vi "template-state-machine-basic.vi"() -> ()   [LabVIEW 2024]
uses:
  state-enum.ctl
  utils-sub-vi/csv-file-logging-util/filepath-selection.ctl
  utils-sub-vi/csv-file-logging-util/datalogging-options.ctl
  serial-options.ctl
  sensor-options.ctl
panel:
  out "return count":u32
  out "Bytes at Port":u32
  out "Log File Open":bool
  in  "Tab Control":enum32{"Data", "Settings"}(tab)
  in  "?":dbl(slide) scale=0.0..10.0
  out "Logged CSV out":string
  out "Serial msg":string
  in  "Datalogging options":T1={"data-precision"=3, "Include Date"=FALSE, "Include Timestamp"=TRUE, "Include Milliseconds"=FALSE, "sample-rate (Hz)"=4.0, "Logging Active"=TRUE}
  in  "Log Filepath Selection":T2={"Log Filepath Source"=enum."Application Relative (Auto)", "Log File Path (Manual)"=path "C:/Users/dheard/Documents/0002-labview-projects/adam-4xxx/template/data", "Log File Folder Name"="data", "log file name"="log", "Include Date in Filename"=TRUE, "Include Time in Filename"=TRUE}
  in  "Serial Port Options":T3={"COM Port (COM10)"="COM10", "baud rate (19200)"=19200, "Simulate Hardware"=FALSE} {"baud rate (19200)" max=115200 step=1200}
  in  "Sensor Options":T4={"Display Units"="PSI", "Zero Offset"=2.62, "Sensor Min"=0.0, "Sensor Max"=500.0, "Signal Min"=0.0, "Signal Max"=100.0, "Conversion Factor"=0.0}
  in  "save-settings":bool
  in  "load-settings":bool
  in  "Settings file":path
  out "Sample Rate (Hz)":dbl format="%-#3.3f"
  in  "Debug Mode":bool
  out "Loop Time (mS)":u32
  out "State:":T5
  out "error IO":errorcluster
  in  "stop":bool
  in  "start":bool
  in  "Exit":bool
  # "Template Logger"
  # "Conversion Factor to\nCalculate User Units from Sensor Units"
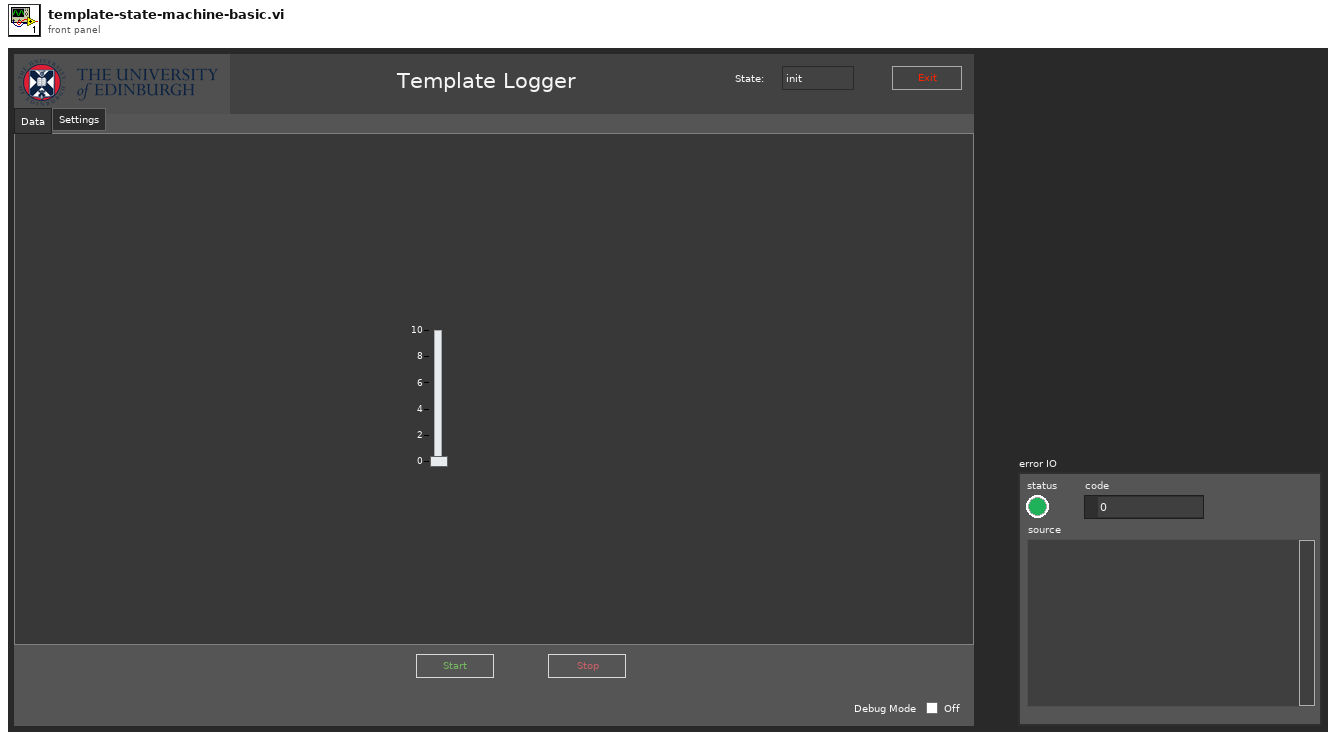
[diagram p1: front panel]
types:
  T1 = typedef "datalogging-options.ctl" = cluster{"data-precision":i32, "Include Date":bool, "Include Timestamp":bool, "Include Milliseconds":bool, "sample-rate (Hz)":dbl, "Logging Active":bool}
  T2 = typedef "filepath-selection.ctl" = cluster{"Log Filepath Source":enum16{"Application Relative (Auto)", "VI Relative (Auto)", "Complete Path (Manual)"}, "Log File Path (Manual)":path, "Log File Folder Name":string, "log file name":string, "Include Date in Filename":bool, "Include Time in Filename":bool}
  T3 = typedef "serial-options.ctl" = cluster{"COM Port (COM10)":refnum<visa-resource-name>, "baud rate (19200)":u32, "Simulate Hardware":bool}
  T4 = typedef "sensor-options.ctl" = cluster{"Display Units":string, "Zero Offset":dbl, "Sensor Min":dbl, "Sensor Max":dbl, "Signal Min":dbl, "Signal Max":dbl, "Conversion Factor":dbl}
  T5 = typedef "state-enum.ctl" = enum16{"init", "recall-settings", "save-settings", "wait", "start", "pre-run", "run", "stop", "shutdown", "exit"}
  T6 = enum8{"Enabled", "Disabled", "Disabled and Grayed Out"}
  T7 = enum16{"open", "replace", "create", "open or create", "replace or create", "replace or create with confirmation"}
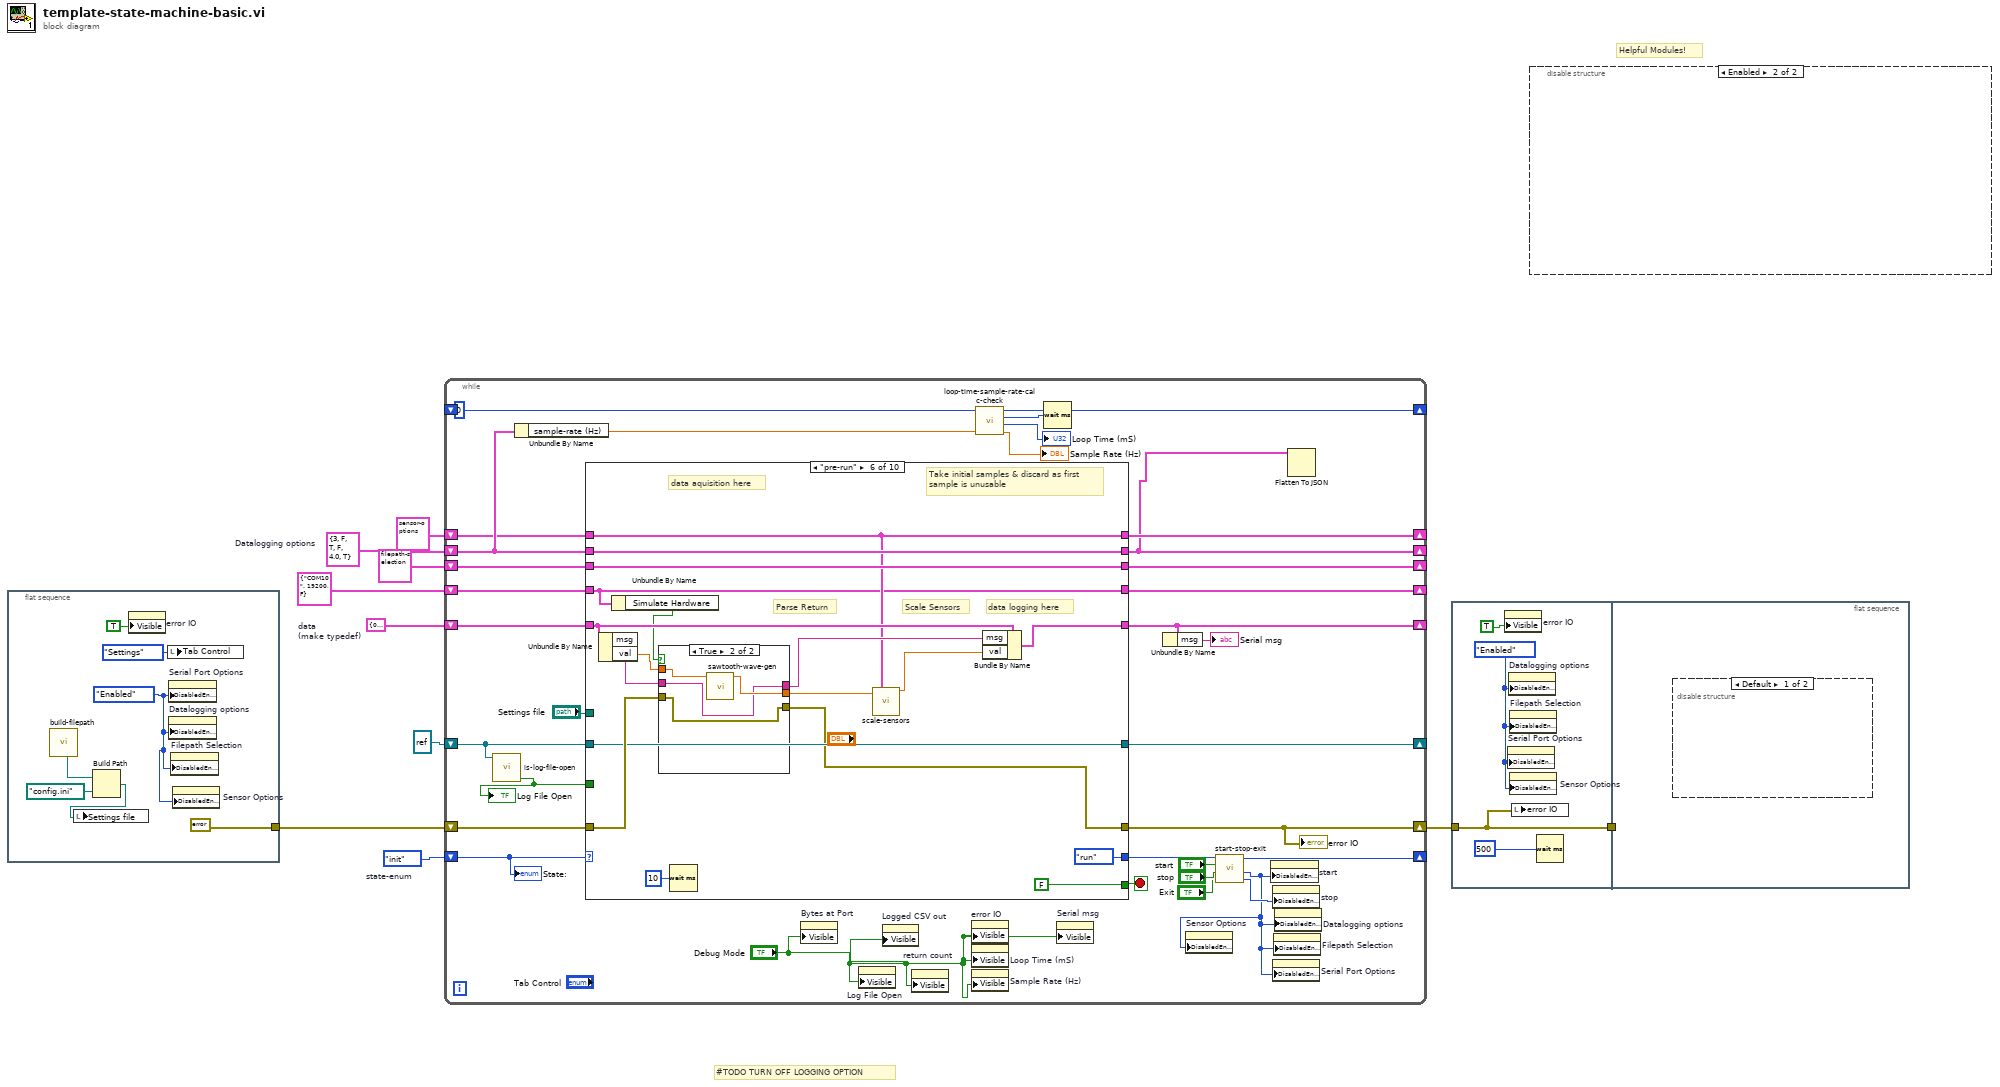
[diagram p0: block diagram]
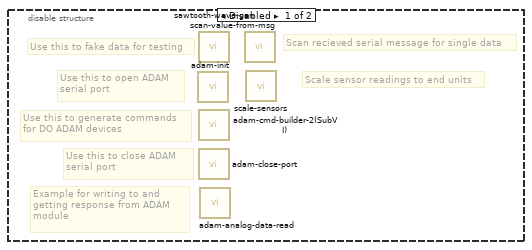
[diagram p2: hidden frame]
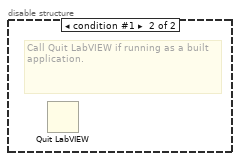
[diagram p3: hidden frame]
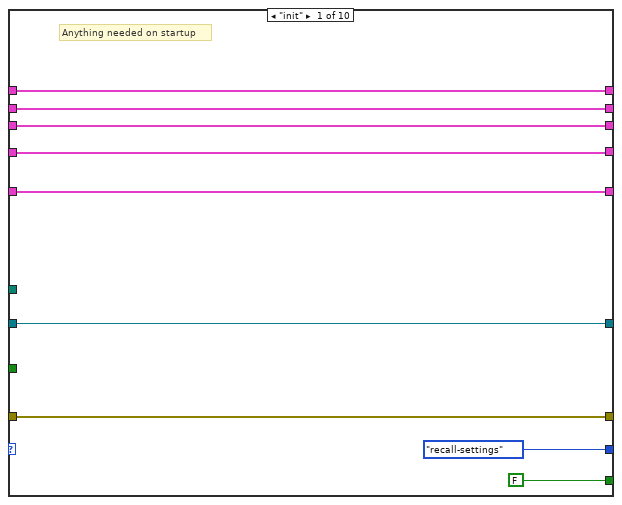
[diagram p4: hidden frame]
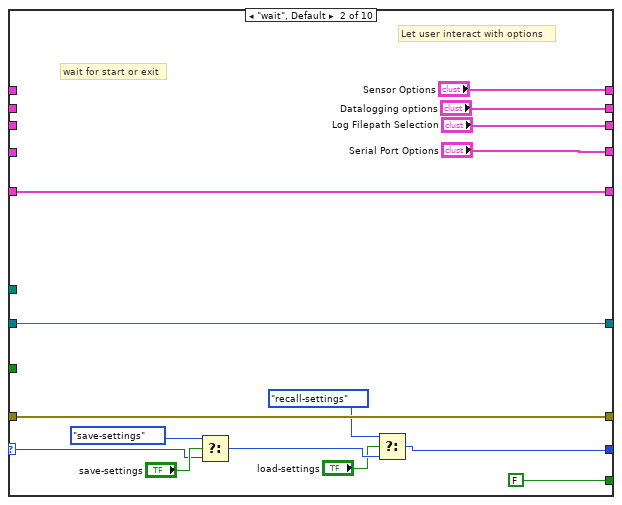
[diagram p5: hidden frame]
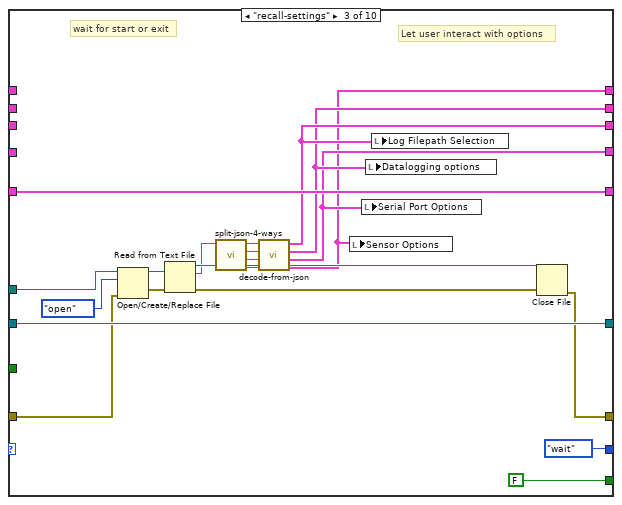
[diagram p6: hidden frame]
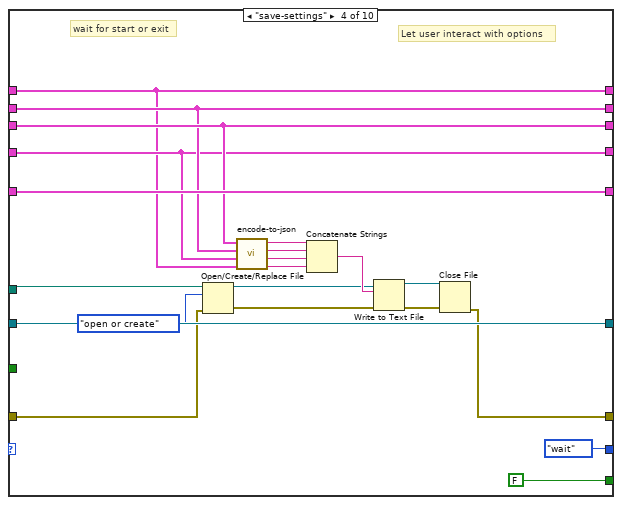
[diagram p7: hidden frame]
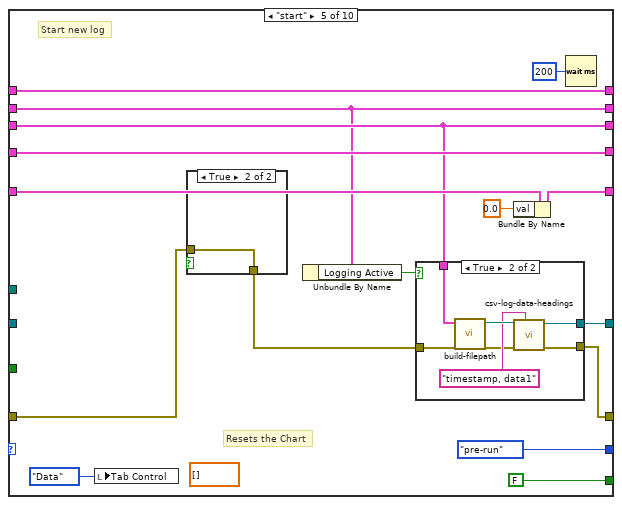
[diagram p8: hidden frame]
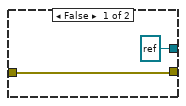
[diagram p10: hidden frame]
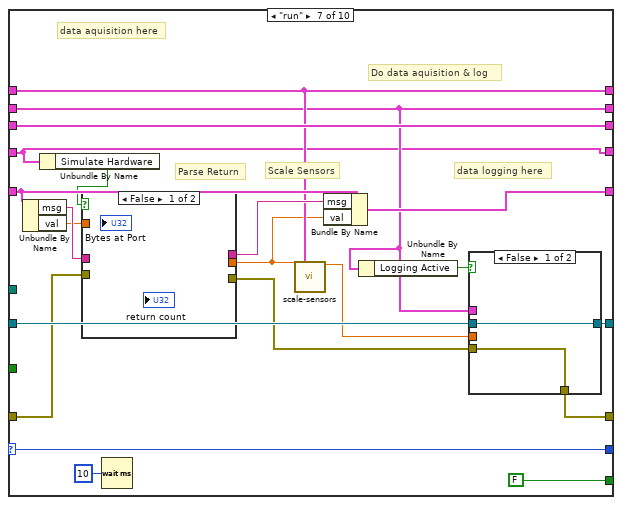
[diagram p12: hidden frame]
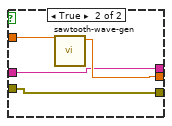
[diagram p13: hidden frame]
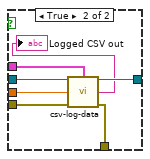
[diagram p14: hidden frame]
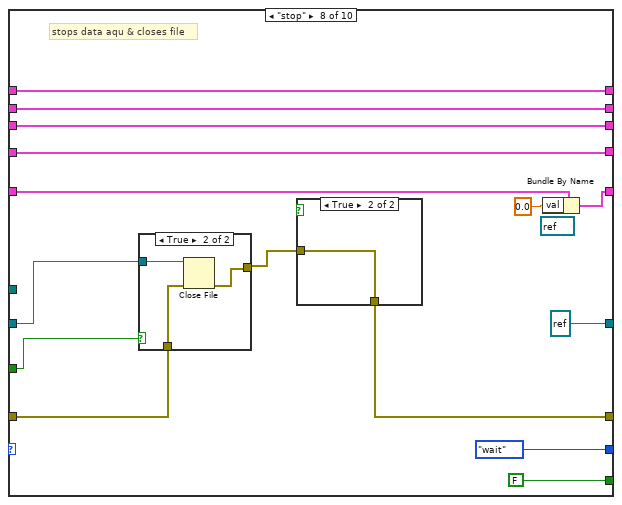
[diagram p15: hidden frame]
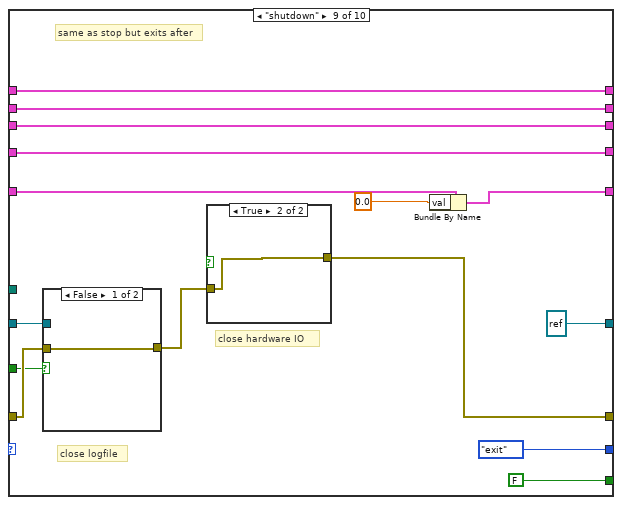
[diagram p18: hidden frame]
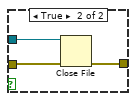
[diagram p20: hidden frame]
diagram:
  w3 = T1 {"data-precision"=3, "Include Date"=FALSE, "Include Timestamp"=TRUE, "Include Milliseconds"=FALSE, "sample-rate (Hz)"=4.0, "Logging Active"=TRUE}  # Datalogging options
  w8 = cluster{"val":dbl, "bool":bool, "msg":string} {"val"=0.0, "bool"=FALSE, "msg"=""}  # data (make typedef)
  w11 = state-enum."init"  # state-enum
  # "#TODO TURN OFF LOGGING OPTION"
  # "Helpful Modules!"
  n1 = flat-sequence {
    tunnel: [errorcluster {"status"=FALSE, "code"=0, "source"=""} ("error IO")] -> w7
    frame #0 {
      w15 = T6."Enabled" ("Disabled")
      n2 = call "build-filepath.vi"() -> ("Application Directory"=w14:path)  [unwired: 9 in, 2 out]
      n3 = Build Path(base path=w14, name or relative path=path "config.ini") -> (appended path=w12:path)
      n4 = local write "Settings file"(w12) -> ()
      n5 = property on="error IO" class="Clust (strict)"("Visible"=TRUE) -> ()  [unwired: 2 in, 2 out]
      n6 = local write "Tab Control"(enum32{"Data", "Settings"}."Settings" ("Tab Control")) -> ()
      n7 = property on="Serial Port Options" class="Clust (strict)"("DisabledEnum"=w15) -> ()  [unwired: 2 in, 2 out]
      n8 = property on="Datalogging options" class="Clust (strict)"("DisabledEnum"=w15) -> ()  [unwired: 2 in, 2 out]
      n9 = property on="Filepath Selection" class="Clust (strict)"("DisabledEnum"=w15) -> ()  [unwired: 2 in, 2 out]
      n10 = property on="Sensor Options" class="Clust (strict)"("DisabledEnum"=w15) -> ()  [unwired: 2 in, 2 out]
    }
  }
  n11 = while {
    shift-right: [w49] -> _
    shift-left: w11 -> [w51]
    shift-right: [w43] -> w9
    shift-left: w7 -> [w44]
    shift-right: [w26] -> _
    shift-left: w8 -> [w42]
    shift-right: [w39] -> _
    shift-left: u32 0 ("millisecond timer value") -> [w41]
    shift-right: [w35] -> _
    shift-left: T2 {"Log Filepath Source"=enum."Application Relative (Auto)", "Log File Path (Manual)"=path "C:/Users/dheard/Documents/0002-labview-projects/ammonia-absorbsion-rig/data", "Log File Folder Name"="data", "log file name"="log", "Include Date in Filename"=TRUE, "Include Time in Filename"=TRUE} ("Filepath Selection") -> [w34]
    shift-right: [w33] -> _
    shift-left: refnum<file> refnum ("Byte Stream File out") -> [w32]
    shift-right: [w20] -> _
    shift-left: w3 -> [w30]
    shift-right: [w27] -> _
    shift-left: T3 {"COM Port (COM10)"="COM10", "baud rate (19200)"=19200, "Simulate Hardware"=FALSE} ("Serial Port Options") -> [w28]
    shift-right: [w24] -> _
    shift-left: T4 {"Display Units"="units", "Zero Offset"=2.62, "Sensor Min"=0.0, "Sensor Max"=500.0, "Signal Min"=0.0, "Signal Max"=100.0, "Conversion Factor"=0.0} ("Sensor Options") -> [w22]
    stop <- w45 stop-if-true
    n12 = call "is-log-file-open.vi"("Byte Stream File in"=w32) -> ("Log File Open"=w31:bool)  [unwired: 10 in]
    "Log File Open" <- w31
    n13 = Unbundle By Name(w30) -> ("sample-rate (Hz)"=w29:dbl)
    n14 = case shown="\"pre-run\"" w51 {
      selector: w51 -> [_ w66 _ _ _ _ w185 _ _ _]
      tunnel: [state-enum."recall-settings" w61 state-enum."wait" state-enum."wait" state-enum."pre-run" state-enum."run" w185 state-enum."wait" state-enum."exit" state-enum."exit"] -> w50
      tunnel: [FALSE FALSE FALSE FALSE FALSE FALSE FALSE FALSE FALSE TRUE] -> w45
      tunnel: [w58 w74 w86 w97 w127 w149 w180 w202 w222 w248] -> w43
      tunnel: w44 -> [w58 w74 w90 w103 w124 w157 w179 w207 w228 w248]
      tunnel: [w57 w73 w95 w116 w130 w160 w184 w210 w231 w247] -> w26
      tunnel: w42 -> [w57 w73 w95 w116 w131 w155 w177 w212 w233 w247]
      tunnel: [w55 "Log Filepath Selection" w79 w110 w120 w159 w181 w206 w227 w245] -> w35
      tunnel: w34 -> [w55 _ _ w110 w120 w159 w181 w206 w227 w245]
      tunnel: [w56 w71 w94 w115 w128 w150 w182 refnum<file> refnum ("log file Byte Stream File out") refnum<file> refnum ("log file Byte Stream File out") w246] -> w33
      tunnel: w32 -> [w56 w71 w94 w115 _ w150 w183 w209 w230 w246]
      tunnel: [w54 "Datalogging options" w78 w109 w119 w158 w171 w205 w226 w244] -> w20
      tunnel: w30 -> [w54 _ _ w109 w119 w158 w171 w205 w226 w244]
      tunnel: w31 -> [_ _ _ _ _ _ _ w200 w225 _]
      tunnel: w28 -> [w53 _ _ w108 w125 w146 w169 w204 w224 w243]
      tunnel: [w53 "Serial Port Options" w77 w108 w125 w146 w169 w204 w224 w243] -> w27
      tunnel: [w52 "Sensor Options" w76 w107 w122 w152 w173 w201 w221 w242] -> w24
      tunnel: w22 -> [w52 _ _ w107 w122 w152 w173 w201 w221 w242]
      tunnel: "Settings file" -> [_ _ w92 w98 _ _ _ _ _ _]
      frame "init" {
        # "Anything needed on startup"
      }
      frame "wait", Default {
        # "Let user interact with options"
        # "wait for start or exit"
        n15 = Select(t=state-enum."save-settings", s="save-settings", f=w66) -> (s? t:f=w64:T5)
        n16 = Select(t=state-enum."recall-settings", s="load-settings", f=w64) -> (s? t:f=w61:T5)
      }
      frame "recall-settings" {
        # "Let user interact with options"
        # "wait for start or exit"
        n17 = Open/Create/Replace File(file path (use dialog)=w92, error in=w90, operation (0:open)=T7."open") -> (refnum out=w89:refnum<file>, error out=w88:errorcluster)  [unwired: 3 in, 1 out]
        n18 = Read from Text File(file (use dialog)=w89, error in=w88) -> (refnum out=w85:refnum<file>, text=w84:string, error out=w87:errorcluster)  [unwired: 2 in, 1 out]
        n19 = call "split-json-4-ways.vi"("json-string-in"=w84) -> ("sensor-json"=w80:string, "serial-json"=w81:string, "datalogging-json"=w82:string, "filepath-json"=w83:string)  [unwired: 7 in]
        n20 = call "decode-from-json.vi"("sensor-options-json"=w80, "serial-port-json"=w81, "data-logging-json"=w82, "filepath-json"=w83) -> ("Sensor Option Recall"=w76:T4, "Serial Port Recall"=w77:T3, "Datalogging Recall"=w78:T1, "Filepath Recall"=w79:T2)  [unwired: 4 in]
        n21 = local write "Sensor Options"(w76) -> ()
        n22 = local write "Serial Port Options"(w77) -> ()
        n23 = local write "Datalogging options"(w78) -> ()
        n24 = local write "Log Filepath Selection"(w79) -> ()
        n25 = Close File(refnum=w85, error in=w87) -> (error out=w86:errorcluster)  [unwired: 1 out]
      }
      frame "save-settings" {
        # "Let user interact with options"
        # "wait for start or exit"
        n26 = Open/Create/Replace File(file path (use dialog)=w98, error in=w103, operation (0:open)=T7."open or create") -> (refnum out=w102:refnum<file>, error out=w101:errorcluster)  [unwired: 3 in, 1 out]
        n27 = call "encode-to-json.vi"("Sensor Options"=w107, "Serial Port Options"=w108, "Datalogging options"=w109, "Filepath Selection"=w110) -> ("sensor-options-json"=w106:string, "serial-port-json"=w111:string, "data-logging-json"=w112:string, "filepath-json"=w113:string)  [unwired: 4 in]
        n28 = Concatenate Strings(w113, w112, w111, w106) -> (w105:string)
        n29 = Write to Text File(file (use dialog)=w102, text=w105, error in=w101) -> (refnum out=w100:refnum<file>, error out=w99:errorcluster)  [unwired: 1 in, 1 out]
        n30 = Close File(refnum=w100, error in=w99) -> (error out=w97:errorcluster)  [unwired: 1 out]
      }
      frame "start" {
        (unwired) dbl[] [] ("History Data")
        # "Start new log"
        # "Resets the Chart"
        n31 = local write "Tab Control"(enum32{"Data", "Settings"}."Data" ("Tab Control")) -> ()
        n32 = case shown="True" {
          selector: _ -> [_ _]
          tunnel: w124 -> [w134 w135]
          tunnel: [w134 w135] -> w123
          frame False {
          }
          frame True {
          }
        }
        n33 = Unbundle By Name(w119) -> ("Logging Active"=w118:bool)
        n34 = case shown="True" w118 {
          tunnel: [refnum<file> refnum ("Byte Stream File out") w141] -> w128
          tunnel: [w136 w140] -> w127
          tunnel: w123 -> [w136 w139]
          tunnel: w120 -> [_ w138]
          frame False {
          }
          frame True {
            n35 = call "build-filepath.vi"("Filepath Selection"=w138) -> ("appended path for log file"=w143:path)  [unwired: 8 in, 2 out]
            n36 = call "csv-log-data-headings.vi"("CSV Data Headings"="timestamp, data1", "error in (no error)"=w139, "Log File Path"=w143) -> ("error out"=w140:errorcluster, "Byte Stream File out"=w141:refnum<file>)  [unwired: 6 in, 1 out]
          }
        }
        n37 = Bundle By Name(cluster=w131, "val"=0.0 ("output")) -> (w130:cluster{"val":dbl, "bool":bool, "msg":string})
        n38 = Wait (ms)(milliseconds to wait=u32 200) -> ()  [unwired: 1 out]
      }
      frame "pre-run" {
        # "Take initial samples & discard as first\nsample is unusable"
        # "Scale Sensors"
        # "Parse Return"
        # "data logging here"
        # "data aquisition here"
        n39 = Unbundle By Name(w155) -> ("msg"=w154:string, "val"=w144:dbl)
        n40 = Unbundle By Name(w146) -> ("Simulate Hardware"=w145:bool)
        n41 = case shown="True" w145 {
          tunnel: w157 -> [_ w162]
          tunnel: w154 -> [_ w163]
          tunnel: [_ w163] -> w153
          tunnel: [_ w164] -> w151
          tunnel: [_ w162] -> w149
          tunnel: w144 -> [_ w165]
          frame False {
          }
          frame True {
            n42 = call "sawtooth-wave-gen.vi"("current-val"=w165) -> ("output"=w164:dbl)  [unwired: 10 in]
          }
        }
        n43 = Wait (ms)(milliseconds to wait=u32 10) -> ()  [unwired: 1 out]
        n44 = call "scale-sensors.vi"("Measured Value (mV)"=w151, "Sensor Options"=w152) -> ("Calculated Value (User Specified Unit)"=w147:dbl)  [unwired: 8 in, 5 out]
        n45 = Bundle By Name(cluster=w155, "msg"=w153, "val"=w147) -> (w160:cluster{"val":dbl, "bool":bool, "msg":string})
      }
      frame "run" {
        # "Scale Sensors"
        # "Parse Return"
        # "data logging here"
        # "data aquisition here"
        # "Do data aquisition & log"
        n46 = Unbundle By Name(w177) -> ("msg"=w176:string, "val"=w167:dbl)
        n47 = Unbundle By Name(w169) -> ("Simulate Hardware"=w168:bool)
        n48 = case shown="False" w168 {
          tunnel: w179 -> [_ w190]
          tunnel: w176 -> [_ w187]
          tunnel: [_ w190] -> w175
          tunnel: [_ w187] -> w174
          tunnel: [_ w188] -> w166
          tunnel: w167 -> [_ w189]
          frame False {
          }
          frame True {
            n49 = call "sawtooth-wave-gen.vi"("current-val"=w189) -> ("output"=w188:dbl)  [unwired: 10 in]
          }
        }
        n50 = Wait (ms)(milliseconds to wait=u32 10) -> ()  [unwired: 1 out]
        n51 = call "scale-sensors.vi"("Measured Value (mV)"=w166, "Sensor Options"=w173) -> ("Calculated Value (User Specified Unit)"=w172:dbl)  [unwired: 8 in, 5 out]
        n52 = Bundle By Name(cluster=w177, "msg"=w174, "val"=w166) -> (w184:cluster{"val":dbl, "bool":bool, "msg":string})
        n53 = Unbundle By Name(w171) -> ("Logging Active"=w170:bool)
        n54 = case shown="False" w170 {
          tunnel: w183 -> [w192 w199]
          tunnel: [w192 w198] -> w182
          tunnel: [w191 w196] -> w180
          tunnel: w171 -> [_ w195]
          tunnel: w175 -> [w191 w194]
          tunnel: w172 -> [_ w193]
          frame False {
          }
          frame True {
            n55 = call "csv-log-data.vi"("log file Byte Stream File in"=w199, "Datalogging options"=w195, "Data Point In"=w193, "error in (no error)"=w194) -> ("log file Byte Stream File out"=w198:refnum<file>, "Logged CSV out"=→"Logged CSV out":string, "error out"=w196:errorcluster)  [unwired: 7 in, 2 out]
          }
        }
      }
      frame "stop" {
        (unwired) refnum<visa-resource-name> refnum ("VISA resource name out")
        # "stops data aqu & closes file"
        n56 = case shown="True" w200 {
          tunnel: w209 -> [_ w220]
          tunnel: w207 -> [w217 w219]
          tunnel: [w217 w218] -> w203
          frame False {
          }
          frame True {
            n57 = Close File(refnum=w220, error in=w219) -> (error out=w218:errorcluster)  [unwired: 1 out]
          }
        }
        n58 = case shown="True" {
          selector: _ -> [_ _]
          tunnel: w203 -> [w215 w216]
          tunnel: [w215 w216] -> w202
          frame False {
          }
          frame True {
          }
        }
        n59 = Bundle By Name(cluster=w212, "val"=0.0 ("output")) -> (w210:cluster{"val":dbl, "bool":bool, "msg":string})
      }
      frame "shutdown" {
        # "close hardware IO"
        # "close logfile"
        # "same as stop but exits after"
        n60 = case shown="False" w225 {
          tunnel: w230 -> [_ w241]
          tunnel: w228 -> [w238 w240]
          tunnel: [w238 w239] -> w223
          frame False {
          }
          frame True {
            n61 = Close File(refnum=w241, error in=w240) -> (error out=w239:errorcluster)  [unwired: 1 out]
          }
        }
        n62 = case shown="True" {
          selector: _ -> [_ _]
          tunnel: w223 -> [w236 w237]
          tunnel: [w236 w237] -> w222
          frame False {
          }
          frame True {
          }
        }
        n63 = Bundle By Name(cluster=w233, "val"=0.0 ("output")) -> (w231:cluster{"val":dbl, "bool":bool, "msg":string})
      }
      frame "exit" {
        # "Exit safely"
      }
    }
    "error IO" <- w43
    n64 = property on="Bytes at Port" class="DigNum (strict)"("Visible"="Debug Mode") -> ()  [unwired: 2 in, 2 out]
    n65 = property on="Log File Open" class="Bool (strict)"("Visible"="Debug Mode") -> ()  [unwired: 2 in, 2 out]
    n66 = property on="Logged CSV out" class="Str"("Visible"="Debug Mode") -> ()  [unwired: 2 in, 2 out]
    n67 = property on="return count" class="DigNum (strict)"("Visible"="Debug Mode") -> ()  [unwired: 2 in, 2 out]
    n68 = property on="error IO" class="Clust (strict)"("Visible"="Debug Mode") -> ()  [unwired: 2 in, 2 out]
    n69 = property on="Loop Time (mS)" class="DigNum (strict)"("Visible"="Debug Mode") -> ()  [unwired: 2 in, 2 out]
    n70 = property on="Sample Rate (Hz)" class="DigNum (strict)"("Visible"="Debug Mode") -> ()  [unwired: 2 in, 2 out]
    n71 = call "loop-time-sample-rate-calc-check.vi"("sample-rate-Hz"=w29, "millisecond timer value in"=w41) -> ("Loop Hz"=→"Sample Rate (Hz)":dbl, "Loop Time (mS)"=→"Loop Time (mS)":u32, "sample-rate-delay-mS"=w36:u32, "millisecond timer value out"=w39:u32)  [unwired: 6 in]
    n72 = Wait (ms)(milliseconds to wait=w36) -> ()  [unwired: 1 out]
    n73 = property on="Serial msg" class="Str"("Visible"="Debug Mode") -> ()  [unwired: 2 in, 2 out]
    n74 = Unbundle By Name(w26) -> ("msg"=→"Serial msg":string)
    n75 = call "start-stop-exit.vi"("Exit"="Exit", "stop"="stop", "start"="start", "current-state"=w50) -> ("stop-enable"=w40:T6, "start-enable"=w23:T6, "new-state"=w49:T5)  [unwired: 5 in]
    n76 = property on="Sensor Options" class="Clust (strict)"("DisabledEnum"=w23) -> ()  [unwired: 2 in, 2 out]
    n77 = property on="start" class="Bool"("DisabledEnum"=w23) -> ()  [unwired: 2 in, 2 out]
    n78 = property on="stop" class="Bool"("DisabledEnum"=w40) -> ()  [unwired: 2 in, 2 out]
    n79 = property on="Serial Port Options" class="Clust (strict)"("DisabledEnum"=w23) -> ()  [unwired: 2 in, 2 out]
    n80 = property on="Filepath Selection" class="Clust (strict)"("DisabledEnum"=w23) -> ()  [unwired: 2 in, 2 out]
    n81 = property on="Datalogging options" class="Clust (strict)"("DisabledEnum"=w23) -> ()  [unwired: 2 in, 2 out]
    n82 = Flatten To JSON(anything=w20) -> ()  [unwired: 2 in, 2 out]
    "State:" <- w51
  }
  n83 = flat-sequence {
    tunnel: [w252] -> w10
    tunnel: w9 -> [w252]
    tunnel: w10 -> [_]
    frame #0 {
      w251 = T6."Enabled" ("Disabled")
      n84 = property on="error IO" class="Clust (strict)"("Visible"=TRUE) -> ()  [unwired: 2 in, 2 out]
      n85 = property on="Serial Port Options" class="Clust (strict)"("DisabledEnum"=w251) -> ()  [unwired: 2 in, 2 out]
      n86 = property on="Datalogging options" class="Clust (strict)"("DisabledEnum"=w251) -> ()  [unwired: 2 in, 2 out]
      n87 = property on="Filepath Selection" class="Clust (strict)"("DisabledEnum"=w251) -> ()  [unwired: 2 in, 2 out]
      n88 = property on="Sensor Options" class="Clust (strict)"("DisabledEnum"=w251) -> ()  [unwired: 2 in, 2 out]
      n89 = local write "error IO"(w252) -> ()
      n90 = Wait (ms)(milliseconds to wait=u32 500) -> ()  [unwired: 1 out]
    }
    frame #1 {
      n91 = disable-structure "Conditional Disable Structure" shown="Default" {
        frame condition #0 (active) {
        }
        frame condition #1 {
          # "Call Quit LabVIEW if running as a built application."
          n92 = Quit LabVIEW() -> ()  [unwired: 1 in]
        }
      }
    }
  }
  n93 = disable-structure shown="Enabled" {
    frame Disabled {
      # "Scale sensor readings to end units"
      # "Scan recieved serial message for single data"
      # "Example for writing to and\ngetting response from ADAM\nmodule"
      # "Use this to open ADAM\nserial port"
      # "Use this to close ADAM \nserial port"
      # "Use this to generate commands\nfor DO ADAM devices"
      # "Use this to fake data for testing"
      n94 = call "adam-init.vi"() -> ()  [unwired: 10 in, 2 out]
      n95 = call "sawtooth-wave-gen.vi"() -> ()  [unwired: 11 in, 1 out]
      n96 = call "adam-cmd-builder-2(SubVI).vi"() -> ()  [unwired: 6 in, 6 out]
      n97 = call "adam-close-port.vi"() -> ()  [unwired: 11 in, 1 out]
      n98 = call "adam-analog-data-read.vi"() -> ()  [unwired: 7 in, 5 out]
      n99 = call "scan-value-from-msg.vi"() -> ()  [unwired: 9 in, 3 out]
      n100 = call "scale-sensors.vi"() -> ()  [unwired: 10 in, 6 out]
    }
    frame Enabled {
    }
  }
